vi "Create JSON Schema Interactive.vi"(8 "error in (no error)":errorcluster, 10 "Variant":variant, 11 "JSON Schema in":string) -> (0 "error out":errorcluster, 3 "JSON Schema":string)   [LabVIEW 2019, in "JSON-Schema.lvlib"]
uses:
  JSON-Schema.lvlib
  <vilib>/JDP Science/JSONtext/JSONtext.lvlib
panel:
  in  "ctl path":path
  in  "OK":bool
  in  "Table":string[][](table)
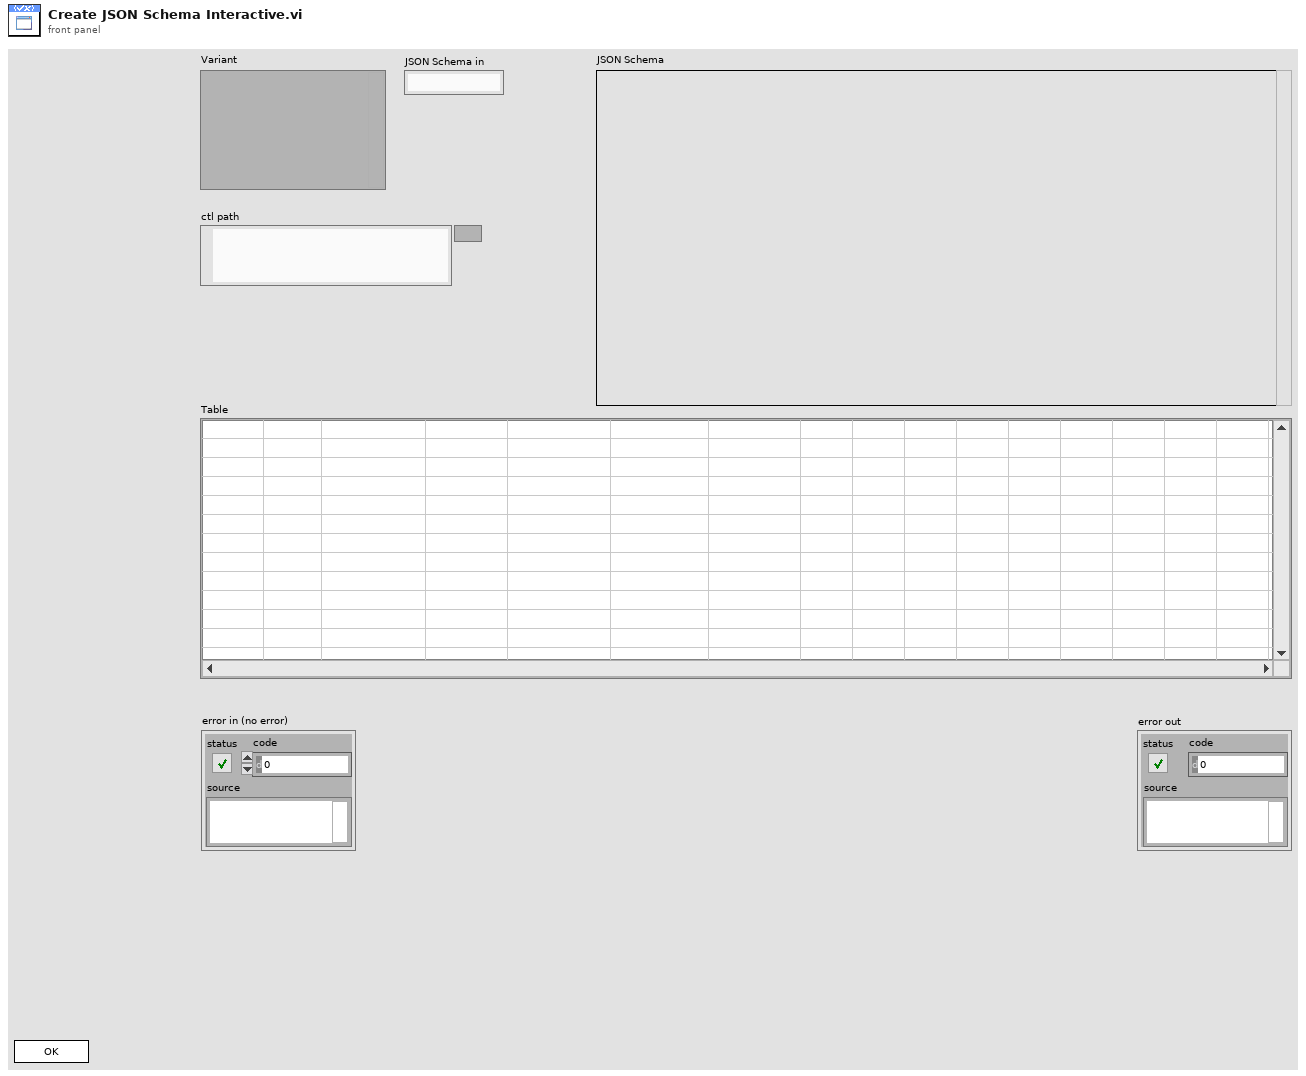
[diagram p1: front panel]
types:
  T1 = enum32{"Invalid", "Standard", "Closed", "Hidden", "Minimized", "Maximized"}
  T2 = enum32{"invalid app kind", "Development System", "Run Time System", "Student Edition", "Embedded LabVIEW", "Evaluation", "Custom"}
  T3 = cluster{"Core":cluster{"Current VI Reference":refnum<vi>, "Close Panel on Exit?":bool}, "Your Boolean data":bool, "Your string data":string}
  T4 = cluster{"Current VI Reference":refnum<vi>, "Close Panel on Exit?":bool}
  T5 = enum32{"Bad", "Idle", "Run top level", "Running"}
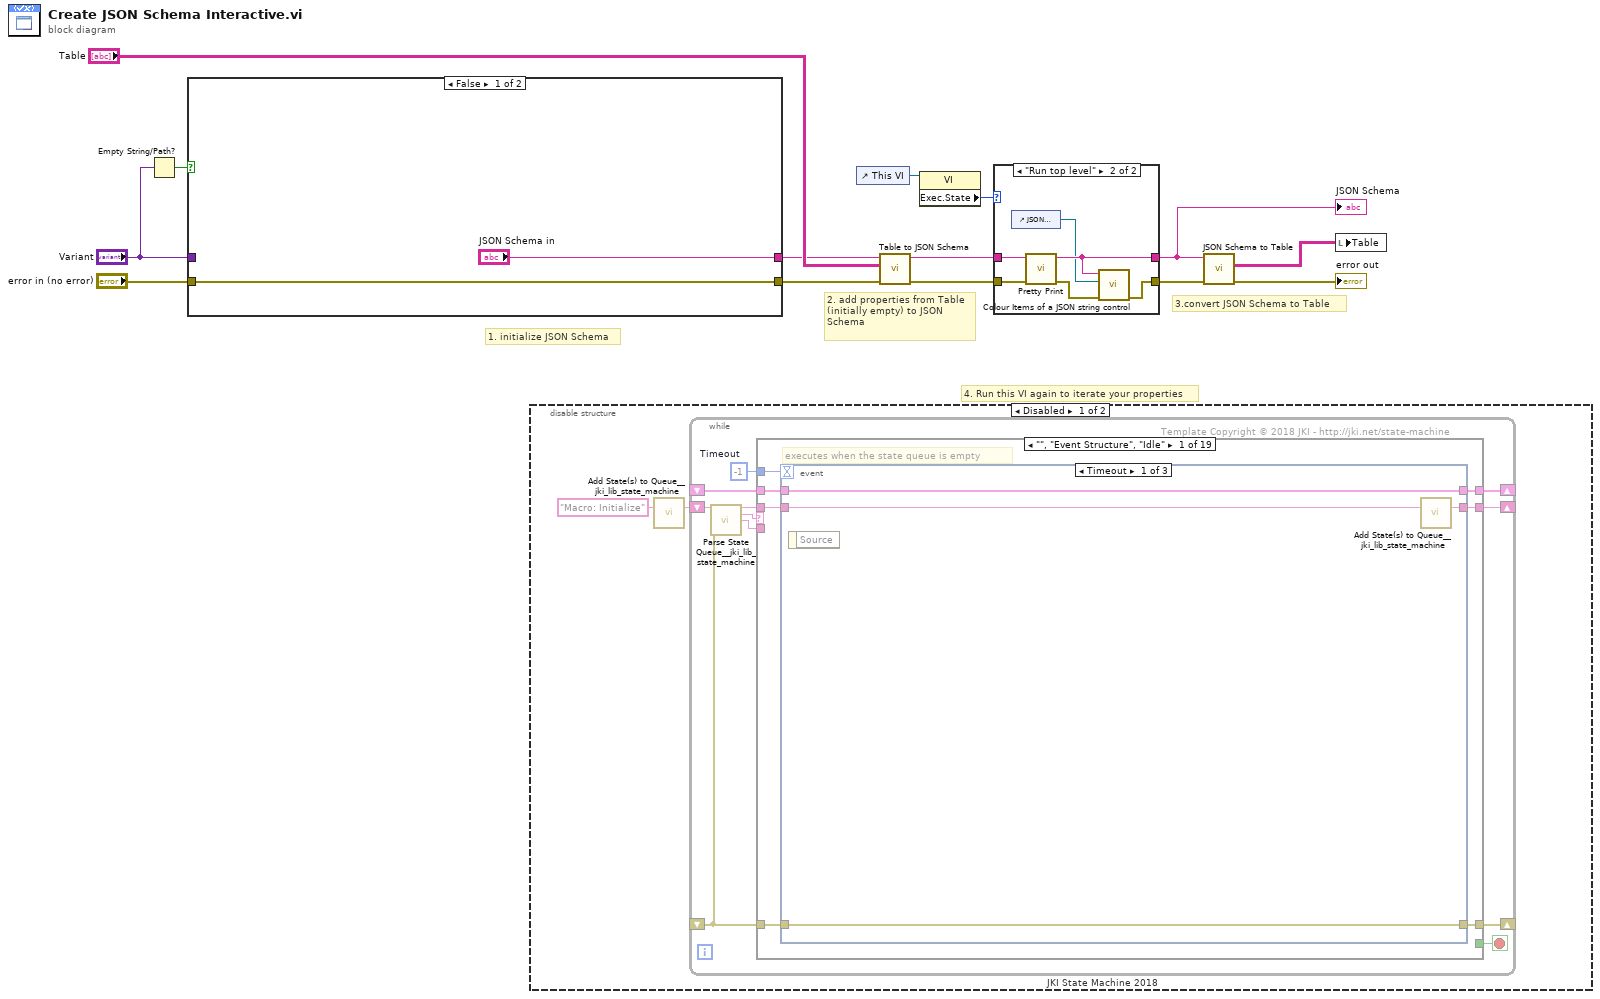
[diagram p0: block diagram]
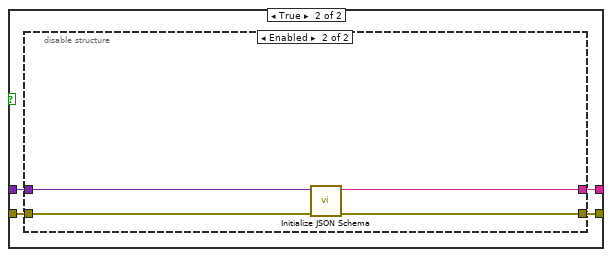
[diagram p2: hidden frame]
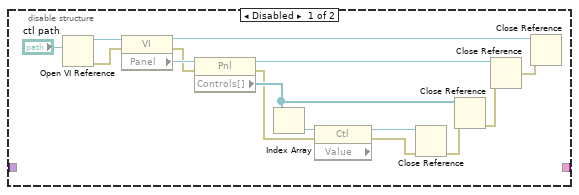
[diagram p3: hidden frame]
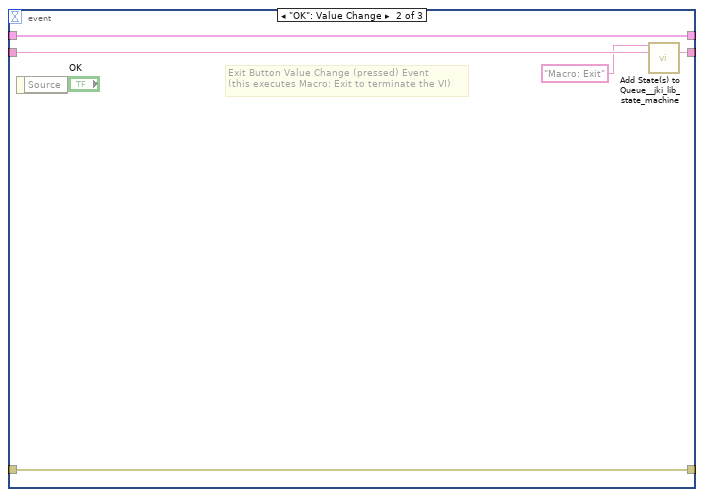
[diagram p5: hidden frame]
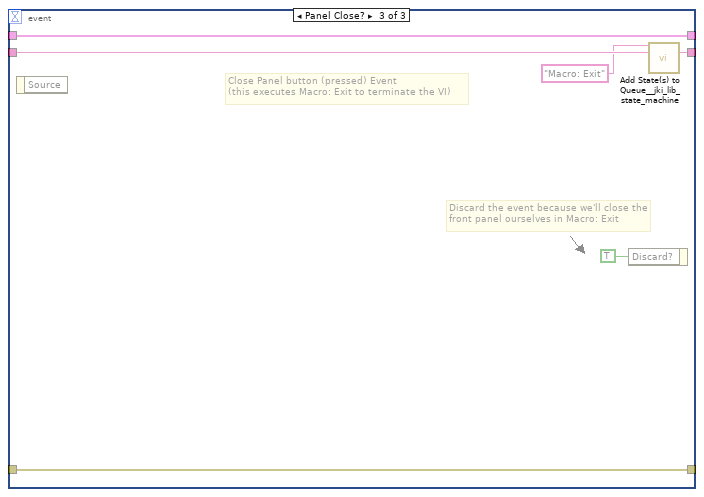
[diagram p6: hidden frame]
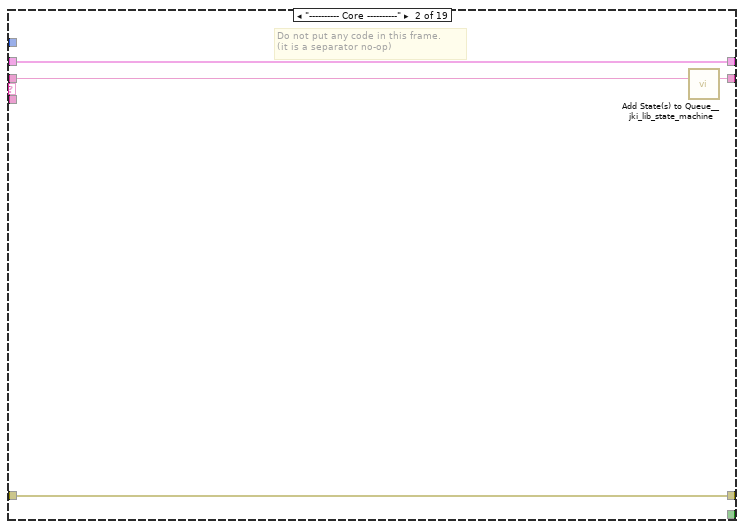
[diagram p7: hidden frame]
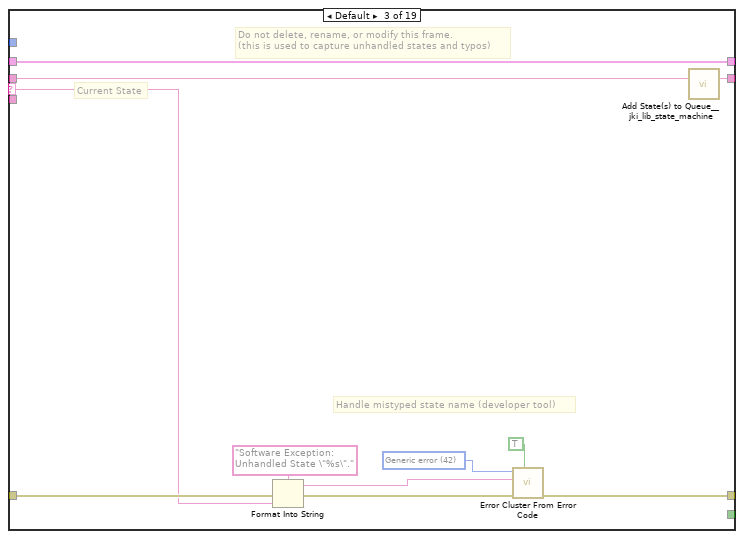
[diagram p8: hidden frame]
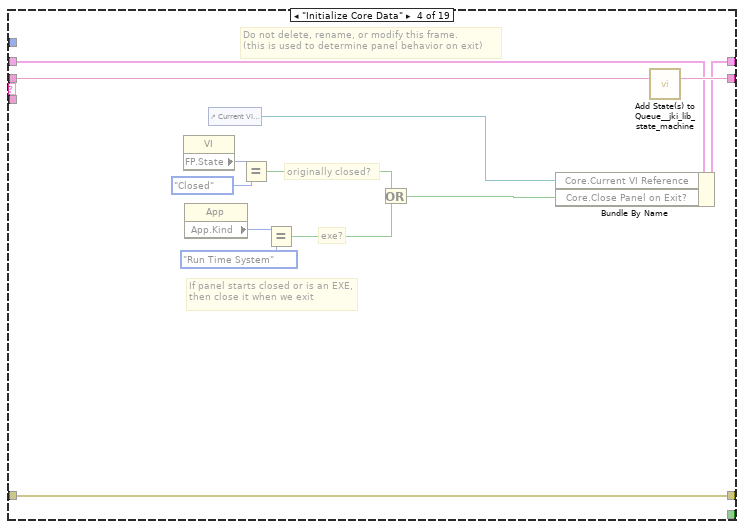
[diagram p9: hidden frame]
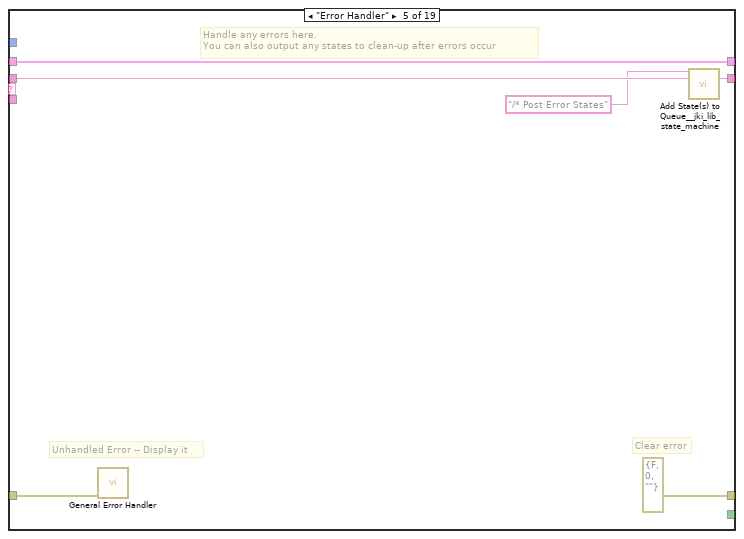
[diagram p10: hidden frame]
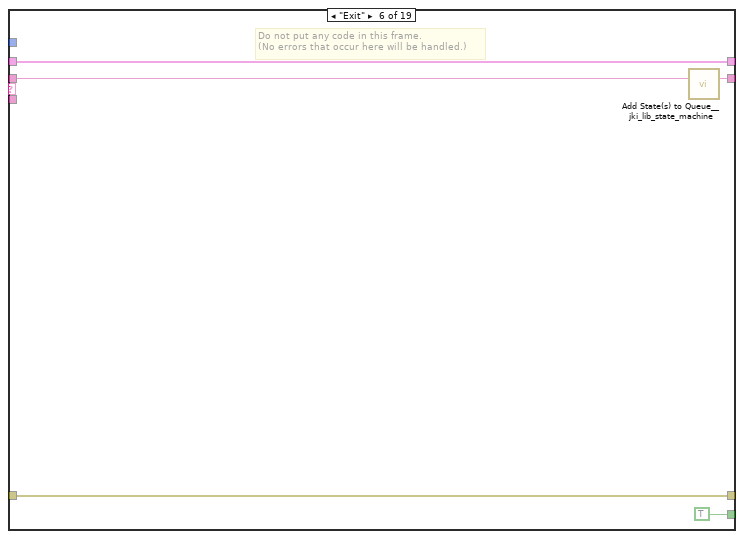
[diagram p11: hidden frame]
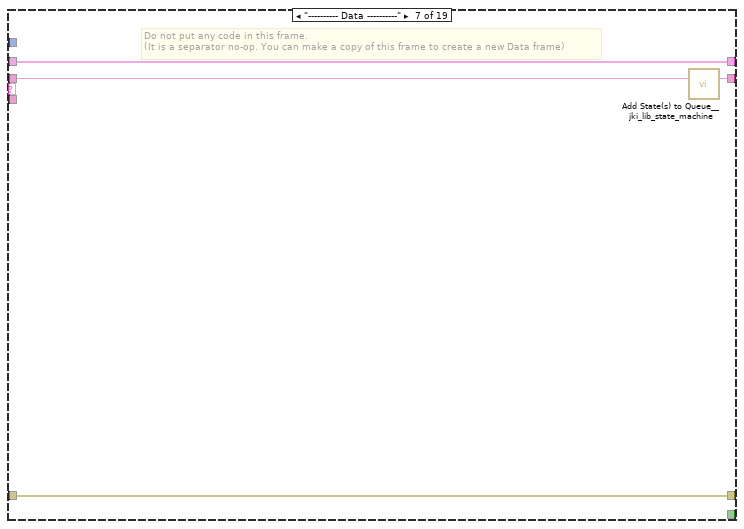
[diagram p12: hidden frame]
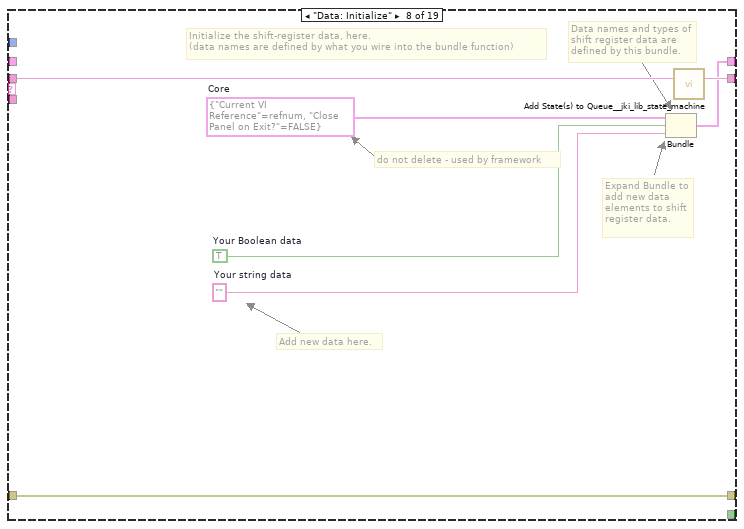
[diagram p13: hidden frame]
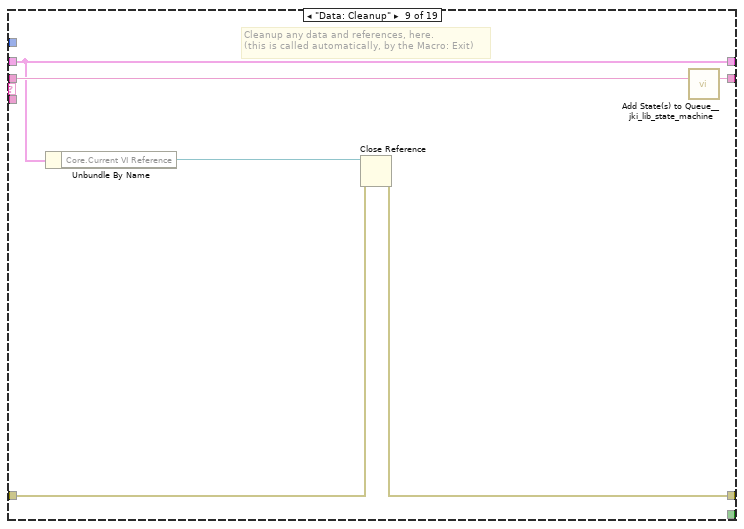
[diagram p14: hidden frame]
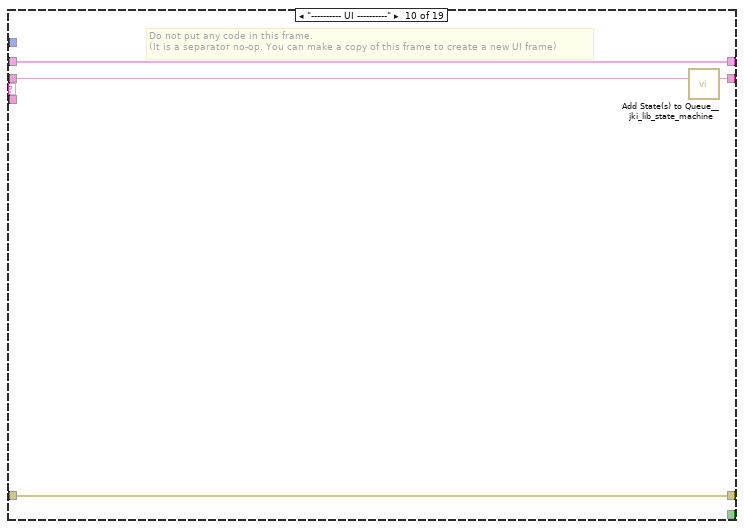
[diagram p15: hidden frame]
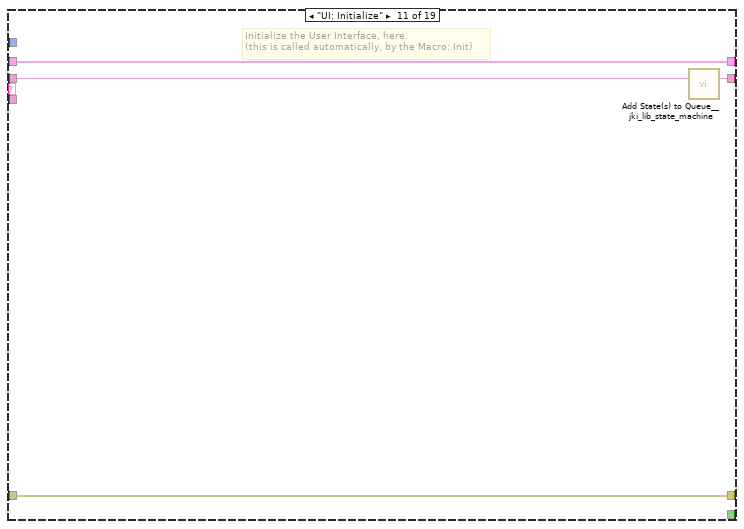
[diagram p16: hidden frame]
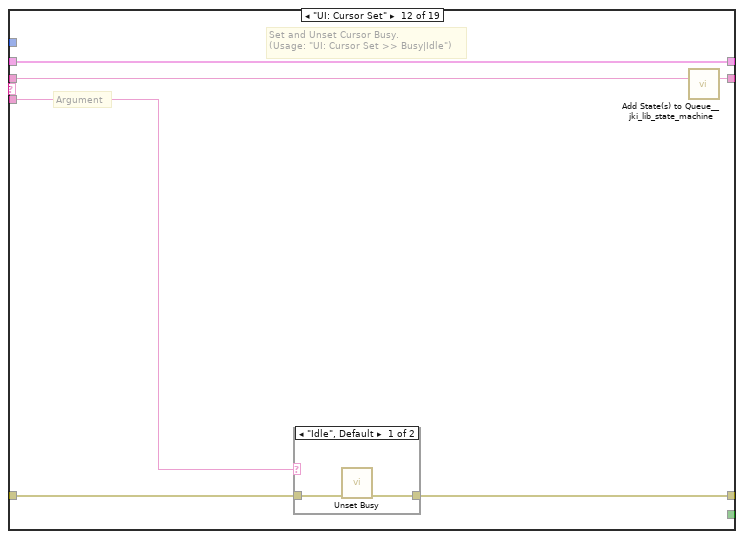
[diagram p17: hidden frame]
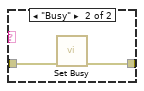
[diagram p18: hidden frame]
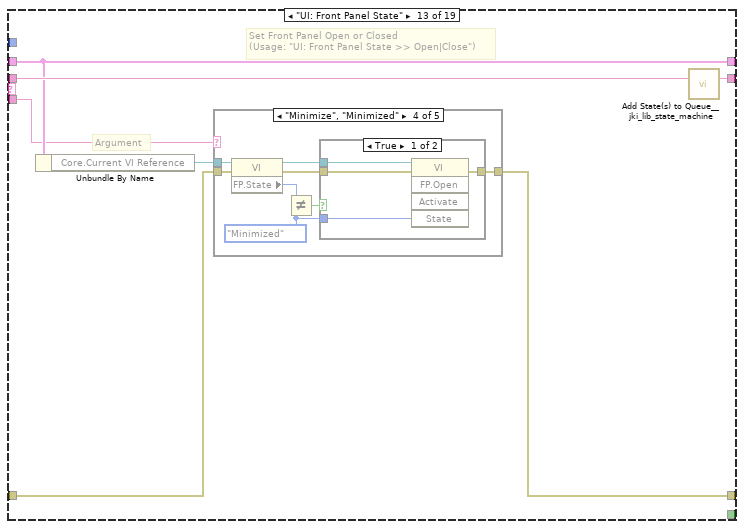
[diagram p19: hidden frame]
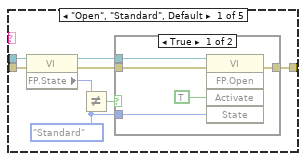
[diagram p20: hidden frame]
diagram:
  # "4. Run this VI again to iterate your properties"
  # "3.convert JSON Schema to Table"
  # "2. add properties from Table (initially empty) to JSON Schema"
  # "1. initialize JSON Schema"
  n1 = Empty String/Path?(string/path="Variant") -> (empty?=w5:bool)
  n2 = case shown="False" w5 {
    tunnel: ["JSON Schema in" w20] -> w1
    tunnel: "Variant" -> [_ w19]
    tunnel: "error in (no error)" -> [w16 w18]
    tunnel: [w16 w17] -> w2
    frame False {
    }
    frame True {
      n3 = disable-structure shown="Enabled" {
        disable-tunnel: [_ w40] -> w20
        disable-tunnel: w19 -> [_ w39]
        disable-tunnel: w18 -> [_ w38]
        disable-tunnel: [_ w37] -> w17
        frame Disabled {
          n4 = Open VI Reference(vi path="ctl path") -> (vi reference=w30:refnum<vi>, error out=w32:errorcluster)  [unwired: 5 in]
          n5 = property class="VI"(reference=w30, error in=w32) -> (reference out=w31:refnum<vi>, error out=w24:errorcluster, "Panel"=w33:refnum<vi>)
          n6 = property class="Pnl"(reference=w33, error in=w24) -> (reference out=w35:refnum<vi>, error out=w21:errorcluster, "Controls[]"=w36:refnum<vi>[])
          n7 = Index Array(array=w36) -> (element=w34:refnum<vi>)  [unwired: 1 in]
          n8 = property class="Ctl"(reference=w34, error in=w21) -> (reference out=w26:refnum<vi>, error out=w23:errorcluster, "Value"=w22:variant)
          n9 = Close Reference(reference=w26, error in (no error)=w23) -> (error out=w25:errorcluster)
          n10 = Close Reference(reference=w36, error in (no error)=w25) -> (error out=w28:errorcluster)
          n11 = Close Reference(reference=w35, error in (no error)=w28) -> (error out=w27:errorcluster)
          n12 = Close Reference(reference=w31, error in (no error)=w27) -> ()  [unwired: 1 out]
        }
        frame Enabled {
          n13 = call "Initialize JSON Schema.vi"("error in (no error)"=w38, "Variant"=w39) -> ("error out"=w37:errorcluster, "JSON Schema out"=w40:string)  [unwired: 8 in]
        }
      }
    }
  }
  n14 = disable-structure shown="Disabled" {
    frame Disabled {
      n15 = call <vilib>:"Add State(s) to Queue__jki_lib_state_machine.vi"("State(s) in (\"\")"="Macro: Initialize") -> ("States Out"=w42:string)  [unwired: 14 in]
      n16 = while "JKI State Machine 2018" {
        shift-right: [w46] -> _
        shift-left: _ -> [w45]
        shift-right: [w49] -> _
        shift-left: _ -> [w43]
        shift-right: [w48] -> _
        shift-left: w42 -> [w50]
        stop <- w47 stop-if-true
        w44 = -1  # Timeout
        # "Template Copyright © 2018 JKI - http://jki.net/state-machine"
        n17 = call <vilib>:"Parse State Queue__jki_lib_state_machine.vi"("State Queue"=w50, "Error In (no error)"=w43) -> ("Remaining States"=w52:string, "Current State"=w53:string, "Arguments"=w51:string)  [unwired: 11 in]
        n18 = case shown="\"\", \"Event Structure\", \"Idle\"" w53 {
          selector: w53 -> [_ _ w80 _ _ _ _ _ _ _ _ _ _ _ _ _ _ _ _]
          tunnel: w52 -> [w60 w79 w84 w103 w109 w114 w118 w125 w131 w135 w139 w145 w156 w225 w230 w240 w244 w248 w252]
          tunnel: w51 -> [_ _ _ _ _ _ _ _ _ _ _ w140 w150 _ _ _ _ _ _]
          tunnel: w45 -> [w58 w76 w82 w96 w106 w112 w115 _ w126 w132 w137 w143 w152 w222 w227 w237 w241 w245 w249]
          tunnel: [w57 w77 w86 w100 errorcluster {"status"=FALSE, "code"=0, "source"=""} ("error out") w111 w116 w122 w127 w133 w136 w141 w153 w223 w228 w238 w242 w246 w250] -> w49
          tunnel: w43 -> [w56 w77 w85 w100 w105 w111 w116 w122 w128 w133 w136 w142 w154 w223 w228 w238 w242 w246 w250]
          tunnel: [w59 w78 w83 w102 w108 w113 w117 w124 w130 w134 w138 w144 w155 w224 w229 w239 w243 w247 w251] -> w48
          tunnel: [_ _ _ _ _ TRUE _ _ _ _ _ _ _ _ _ _ _ _ _] -> w47
          tunnel: [w55 w76 w82 w101 w106 w112 w115 w123 w126 w132 w137 w143 w152 w222 w227 w237 w241 w245 w249] -> w46
          tunnel: w44 -> [w54 _ _ _ _ _ _ _ _ _ _ _ _ _ _ _ _ _ _]
          frame "", "Event Structure", "Idle" {
            # "executes when the state queue is empty"
            n19 = event shown="[0] Timeout" {
              selector: _ -> [_ _ _]
              dyn-events: _ -> [_ _ _]
              timeout: w54 -> [_ _ _]
              tunnel: w60 -> [w64 w69 w75]
              tunnel: [w63 w68 w74] -> w59
              tunnel: w58 -> [w61 w66 w72]
              tunnel: [w62 w67 w73] -> w57
              tunnel: w56 -> [w62 w67 w73]
              tunnel: [w61 w66 w72] -> w55
              event Timeout {
                n20 = event-data() -> ()  [unwired: 1 in, 1 out]
                n21 = call <vilib>:"Add State(s) to Queue__jki_lib_state_machine.vi"("State(s) in (\"\")"=w64) -> ("States Out"=w63:string)  [unwired: 14 in]
              }
              event "OK": Value Change {
                # "Exit Button Value Change (pressed) Event\n(this executes Macro: Exit to terminate the VI)"
                n22 = event-data() -> ()  [unwired: 1 in, 1 out]
                n23 = call <vilib>:"Add State(s) to Queue__jki_lib_state_machine.vi"("State(s) in Front (\"\")"="Macro: Exit", "State(s) in (\"\")"=w69) -> ("States Out"=w68:string)  [unwired: 13 in]
              }
              event Panel Close? {
                # "Discard the event because we'll close the front panel ourselves in Macro: Exit"
                # "Close Panel button (pressed) Event\n(this executes Macro: Exit to terminate the VI)"
                n24 = event-data() -> ()  [unwired: 1 in, 1 out]
                n25 = event-data("Discard?"=TRUE) -> ()  [unwired: 1 in, 1 out]
                n26 = call <vilib>:"Add State(s) to Queue__jki_lib_state_machine.vi"("State(s) in Front (\"\")"="Macro: Exit", "State(s) in (\"\")"=w75) -> ("States Out"=w74:string)  [unwired: 13 in]
              }
            }
          }
          frame "---------- Core ----------" {
            # "Do not put any code in this frame.\n(it is a separator no-op)"
            n27 = call <vilib>:"Add State(s) to Queue__jki_lib_state_machine.vi"("State(s) in (\"\")"=w79) -> ("States Out"=w78:string)  [unwired: 14 in]
          }
          frame Default {
            w89 = 42 items=["No error", "Argument error", "Memory is full", "Out of zone", "End of file", "File already open", "Generic file I/O error", "File not found", "File permission error", "Disk is full", "Duplicate path", "Too many files open", "System feature not enabled", "Resource file not found", "Cannot add resource", "Resource not found", "Image not found", "Image memory error", "Pen does not exist", "Config type invalid", "Config token not found", "Config parse error", "Config memory error", "Bad external code format", "Bad external code offset", "External code not present", "Null window", "Destroy window error", "Null menu", "Print aborted", "Bad print record", "Print driver error", "Windows error during printing", "Memory error during printing", "Print dialog error", "Generic print error", "Invalid device refnum", "Device not found", "Device parameter error", "Device unit error", "Cannot open device", "Device call aborted", "Generic error", "Cancelled by user", "Object ID too low", "Object ID too high", "Object not in heap", "Unknown heap", "Unknown object (invalid DefProc)", "Unknown object (DefProc not in table)", "Message out of range", "Invalid (null) method", "Unknown message", "Manager call not supported", "Bad address", "Network operation in progress", "Network operation timed out", "Connection is busy", "Network attribute not supported", "Network error", "Address in use", "System out of memory", "Connection aborted", "Connection refused", "Not connected", "Already connected", "Connection closed", "Initialization error (interapplication manager)", "Bad occurrence", "Wait on unbound occurrence handler", "Occurrence queue overflow", "Datalog type conflict", "Unused", "Unrecognized type (interapplication manager)", "Memory corrupt", "Failed to make temporary DLL", "Old CIN version", "Drag socket not found", "Failed to load drop-object", "Failed to register OLE object", "Failed to release OLE object", "Format specifier type mismatch", "Unknown format specifier", "Too few format specifiers", "Too many format specifiers", "Scan failed", "Newer CIN version", "Error converting to variant", "Runtime menu error", "Password tampered", "Variant attribute not found", "Incompatible variant data type", "Event data is not available", "Event Store is not present", "Occurrence is not found", "Event Queue is not created", "Event info is not available", "Refnum passed is NULL", "Error retrieving Class GUID", "Error retrieving CoClass GUID", "Error retrieving TypeLib GUID.", "Bad built application magic bytes.", "Specific driver is different from the specific driver associated with the Logical Name.", "There is no session opened to the class driver.", "Max Error", "MAX - Error with config objects", "MAX - Error loading configuration", "MAX - Group not supported"]
            # "Current State"
            # "Do not delete, rename, or modify this frame.\n(this is used to capture unhandled states and typos)"
            # "Handle mistyped state name (developer tool)"
            n28 = Format Into String(format string="Software Exception: Unhandled State \"%s\"." ("message"), error in=w85, w80) -> (resulting string=w88:string, error out=w87:errorcluster)  [unwired: 1 in]
            n29 = call <vilib>:"Error Cluster From Error Code.vi"("show call chain? (False)"=TRUE, "error in (no error)"=w87, "error message (\"\")"=w88, "error code (0)"=w89) -> ("error out"=w86:errorcluster)  [unwired: 5 in]
            n30 = call <vilib>:"Add State(s) to Queue__jki_lib_state_machine.vi"("State(s) in (\"\")"=w84) -> ("States Out"=w83:string)  [unwired: 14 in]
          }
          frame "Initialize Core Data" {
            # "Do not delete, rename, or modify this frame.\n(this is used to determine panel behavior on exit)"
            # "originally closed?"
            # "exe?"
            # "If panel starts closed or is an EXE, then close it when we exit"
            n31 = property class="VI"() -> ("FP.State"=w93:T1)  [unwired: 2 in, 2 out]
            n32 = property class="App"() -> ("App.Kind"=w99:T2)  [unwired: 2 in, 2 out]
            n33 = control-ref of="Current VI Reference"() -> (w94:refnum<vi>)
            n34 = Equal?(x=w93, y=T1."Closed" ("Front Panel Window:State")) -> (x = y?=w91:bool)
            n35 = Equal?(x=w99, y=T2."Run Time System" ("Application:Kind")) -> (x = y?=w97:bool)
            n36 = Or(x=w91, y=w97) -> (x .or. y?=w95:bool)
            n37 = Bundle By Name(cluster=w96, "Core.Current VI Reference"=w94, "Core.Close Panel on Exit?"=w95) -> (w101:T3)
            n38 = call <vilib>:"Add State(s) to Queue__jki_lib_state_machine.vi"("State(s) in (\"\")"=w103) -> ("States Out"=w102:string)  [unwired: 14 in]
          }
          frame "Error Handler" {
            # "Unhandled Error -- Display it"
            # "Handle any errors here.\nYou can also output any states to clean-up after errors occur"
            # "Clear error"
            n39 = call <vilib>:"General Error Handler.vi"("error in (no error)"=w105) -> ()  [unwired: 10 in, 5 out]
            n40 = call <vilib>:"Add State(s) to Queue__jki_lib_state_machine.vi"("State(s) in Front (\"\")"="/* Post Error States", "State(s) in (\"\")"=w109) -> ("States Out"=w108:string)  [unwired: 13 in]
          }
          frame "Exit" {
            # "Do not put any code in this frame.\n(No errors that occur here will be handled.)"
            n41 = call <vilib>:"Add State(s) to Queue__jki_lib_state_machine.vi"("State(s) in (\"\")"=w114) -> ("States Out"=w113:string)  [unwired: 14 in]
          }
          frame "---------- Data ----------" {
            # "Do not put any code in this frame.\n(It is a separator no-op. You can make a copy of this frame to create a new Data frame)"
            n42 = call <vilib>:"Add State(s) to Queue__jki_lib_state_machine.vi"("State(s) in (\"\")"=w118) -> ("States Out"=w117:string)  [unwired: 14 in]
          }
          frame "Data: Initialize" {
            w119 = T4 {"Current VI Reference"=refnum, "Close Panel on Exit?"=FALSE}  # Core
            w121 = TRUE  # Your Boolean data
            w120 = ""  # Your string data
            # "do not delete - used by framework"
            # "Expand Bundle to add new data elements to shift register data."
            # "Add new data here."
            # "Data names and types of shift register data are defined by this bundle."
            # "Initialize the shift-register data, here.\n(data names are defined by what you wire into the bundle function)"
            n43 = Bundle("Core"=w119, "Your Boolean data"=w121, "Your string data"=w120) -> (w123:T3)  [unwired: 1 in]
            n44 = call <vilib>:"Add State(s) to Queue__jki_lib_state_machine.vi"("State(s) in (\"\")"=w125) -> ("States Out"=w124:string)  [unwired: 14 in]
          }
          frame "Data: Cleanup" {
            # "Cleanup any data and references, here.\n(this is called automatically, by the Macro: Exit)"
            n45 = Unbundle By Name(w126) -> ("Core.Current VI Reference"=w129:refnum<vi>)
            n46 = Close Reference(reference=w129, error in (no error)=w128) -> (error out=w127:errorcluster)
            n47 = call <vilib>:"Add State(s) to Queue__jki_lib_state_machine.vi"("State(s) in (\"\")"=w131) -> ("States Out"=w130:string)  [unwired: 14 in]
          }
          frame "---------- UI ----------" {
            # "Do not put any code in this frame.\n(It is a separator no-op. You can make a copy of this frame to create a new UI frame)"
            n48 = call <vilib>:"Add State(s) to Queue__jki_lib_state_machine.vi"("State(s) in (\"\")"=w135) -> ("States Out"=w134:string)  [unwired: 14 in]
          }
          frame "UI: Initialize" {
            # "Initialize the User Interface, here.\n(this is called automatically, by the Macro: Init)"
            n49 = call <vilib>:"Add State(s) to Queue__jki_lib_state_machine.vi"("State(s) in (\"\")"=w139) -> ("States Out"=w138:string)  [unwired: 14 in]
          }
          frame "UI: Cursor Set" {
            # "Argument"
            # "Set and Unset Cursor Busy.\n(Usage: \"UI: Cursor Set >> Busy|Idle\")"
            n50 = case shown="\"Idle\", Default" w140 {
              tunnel: w142 -> [w147 w149]
              tunnel: [w146 w148] -> w141
              frame "Idle", Default {
                n51 = call <vilib>:"Unset Busy.vi"("error in (no error)"=w147) -> ("error out"=w146:errorcluster)  [unwired: 10 in]
              }
              frame "Busy" {
                n52 = call <vilib>:"Set Busy.vi"("error in (no error)"=w149) -> ("error out"=w148:errorcluster)  [unwired: 9 in, 1 out]
              }
            }
            n53 = call <vilib>:"Add State(s) to Queue__jki_lib_state_machine.vi"("State(s) in (\"\")"=w145) -> ("States Out"=w144:string)  [unwired: 14 in]
          }
          frame "UI: Front Panel State" {
            # "Argument"
            # "Set Front Panel Open or Closed\n(Usage: \"UI: Front Panel State >> Open|Close\")"
            n54 = Unbundle By Name(w152) -> ("Core.Current VI Reference"=w151:refnum<vi>)
            n55 = case shown="\"Minimize\", \"Minimized\"" w150 {
              tunnel: w154 -> [w162 w177 w188 w201 w214]
              tunnel: [w164 w178 w190 w203 w216] -> w153
              tunnel: w151 -> [w163 w175 w189 w202 w215]
              frame "Open", "Standard", Default {
                w157 = T1."Standard" ("State")
                n56 = property class="VI"(reference=w163, error in=w162) -> (reference out=w160:refnum<vi>, error out=w161:errorcluster, "FP.State"=w159:T1)
                n57 = Not Equal?(x=w159, y=w157) -> (x != y?=w158:bool)
                n58 = case shown="True" w158 {
                  tunnel: [w168 w170] -> w164
                  tunnel: w161 -> [w167 w170]
                  tunnel: w160 -> [w166 _]
                  tunnel: w157 -> [w165 _]
                  frame True {
                    n59 = invoke class="VI" method="FP.Open"(reference=w166, error in=w167, "Activate"=TRUE, "State"=w165) -> (error out=w168:errorcluster)  [unwired: 1 in, 4 out]
                  }
                  frame False {
                  }
                }
              }
              frame "Close", "Closed" {
                n60 = property class="VI"(reference=w175, error in=w177) -> (reference out=w174:refnum<vi>, error out=w176:errorcluster, "FP.State"=w172:T1)
                n61 = Not Equal?(x=w172, y=T1."Closed" ("Front Panel Window:State")) -> (x != y?=w171:bool)
                n62 = case shown="True" w171 {
                  tunnel: [w179 w182] -> w178
                  tunnel: w176 -> [w179 w181]
                  tunnel: w174 -> [_ w180]
                  frame False {
                  }
                  frame True {
                    n63 = invoke class="VI" method="FP.Close"(reference=w180, error in=w181) -> (error out=w182:errorcluster)  [unwired: 1 in, 2 out]
                  }
                }
              }
              frame "Hidden", "Hide" {
                w183 = T1."Hidden" ("State")
                n64 = property class="VI"(reference=w189, error in=w188) -> (reference out=w186:refnum<vi>, error out=w187:errorcluster, "FP.State"=w185:T1)
                n65 = Not Equal?(x=w185, y=w183) -> (x != y?=w184:bool)
                n66 = case shown="True" w184 {
                  tunnel: [w194 w195] -> w190
                  tunnel: w187 -> [w193 w195]
                  tunnel: w186 -> [w192 _]
                  tunnel: w183 -> [w191 _]
                  frame True {
                    n67 = invoke class="VI" method="FP.Open"(reference=w192, error in=w193, "State"=w191) -> (error out=w194:errorcluster)  [unwired: 2 in, 4 out]
                  }
                  frame False {
                  }
                }
              }
              frame "Minimize", "Minimized" {
                w196 = T1."Minimized" ("State")
                n68 = property class="VI"(reference=w202, error in=w201) -> (reference out=w199:refnum<vi>, error out=w200:errorcluster, "FP.State"=w198:T1)
                n69 = Not Equal?(x=w198, y=w196) -> (x != y?=w197:bool)
                n70 = case shown="True" w197 {
                  tunnel: [w207 w208] -> w203
                  tunnel: w200 -> [w206 w208]
                  tunnel: w199 -> [w205 _]
                  tunnel: w196 -> [w204 _]
                  frame True {
                    n71 = invoke class="VI" method="FP.Open"(reference=w205, error in=w206, "State"=w204) -> (error out=w207:errorcluster)  [unwired: 2 in, 4 out]
                  }
                  frame False {
                  }
                }
              }
              frame "Maximize", "Maximized" {
                w209 = T1."Maximized" ("State")
                n72 = property class="VI"(reference=w215, error in=w214) -> (reference out=w212:refnum<vi>, error out=w213:errorcluster, "FP.State"=w211:T1)
                n73 = Not Equal?(x=w211, y=w209) -> (x != y?=w210:bool)
                n74 = case shown="True" w210 {
                  tunnel: [w220 w221] -> w216
                  tunnel: w213 -> [w219 w221]
                  tunnel: w212 -> [w218 _]
                  tunnel: w209 -> [w217 _]
                  frame True {
                    n75 = invoke class="VI" method="FP.Open"(reference=w218, error in=w219, "State"=w217) -> (error out=w220:errorcluster)  [unwired: 2 in, 4 out]
                  }
                  frame False {
                  }
                }
              }
            }
            n76 = call <vilib>:"Add State(s) to Queue__jki_lib_state_machine.vi"("State(s) in (\"\")"=w156) -> ("States Out"=w155:string)  [unwired: 14 in]
          }
          frame "---------- Macro ----------" {
            # "Do not put any code in this frame.\n(It is a separator no-op. You can make a copy of this frame to create a new Macro frame)"
            n77 = call <vilib>:"Add State(s) to Queue__jki_lib_state_machine.vi"("State(s) in (\"\")"=w225) -> ("States Out"=w224:string)  [unwired: 14 in]
          }
          frame "Macro: Initialize" {
            w226 = "Data: Initialize\nInitialize Core Data\nUI: Initialize\nUI: Front Panel State >> Open"  # Data: Initialize Initialize Core Data UI: Initialize UI: Front Panel State >> Open
            # "Initialization Macro\n(This is called once, when the VI starts)"
            n78 = call <vilib>:"Add State(s) to Queue__jki_lib_state_machine.vi"("State(s) in Front (\"\")"=w226, "State(s) in (\"\")"=w230) -> ("States Out"=w229:string)  [unwired: 13 in]
          }
          frame "Macro: Exit" {
            # "Exit Macro\n(This is called once, when the VI exits)"
            n79 = Unbundle By Name(w237) -> ("Core.Close Panel on Exit?"=w236:bool)
            n80 = Select(t="UI: Front Panel State >> Close", s=w236, f="") -> (s? t:f=w233:string)
            n81 = call <vilib>:"Add State(s) to Queue__jki_lib_state_machine.vi"("State(s) in (\"\")"=w233, "State(s) at Back (\"\")"="Data: Cleanup\nExit") -> ("States Out"=w231:string)  [unwired: 13 in]
            n82 = call <vilib>:"Add State(s) to Queue__jki_lib_state_machine.vi"("State(s) in Front (\"\")"=w231, "State(s) in (\"\")"=w240) -> ("States Out"=w239:string)  [unwired: 13 in]
          }
          frame "---------- New Category ----------" {
            # "Template Separator\n(You can make a copy of, or modify, this frame)"
            n83 = call <vilib>:"Add State(s) to Queue__jki_lib_state_machine.vi"("State(s) in (\"\")"=w244) -> ("States Out"=w243:string)  [unwired: 14 in]
          }
          frame "New Category: 1" {
            # "Your code here.\n(You can make a copy of, or modify, this frame)"
            n84 = call <vilib>:"Add State(s) to Queue__jki_lib_state_machine.vi"("State(s) in (\"\")"=w248) -> ("States Out"=w247:string)  [unwired: 14 in]
          }
          frame "New Category: 2" {
            # "Your code here.\n(You can make a copy of, or modify, this frame)"
            n85 = call <vilib>:"Add State(s) to Queue__jki_lib_state_machine.vi"("State(s) in (\"\")"=w252) -> ("States Out"=w251:string)  [unwired: 14 in]
          }
        }
      }
    }
    frame Enabled {
    }
  }
  n86 = control-ref of="This VI"() -> (w14:refnum<vi>)
  n87 = call "Table to JSON Schema.vi"("error in (no error)"=w2, "Table"="Table", "JSON Schema in"=w1) -> ("error out"=w11:errorcluster, "JSON Schema out"=w12:string)  [unwired: 7 in]
  n88 = property class="VI"(reference=w14) -> ("Exec.State"=w13:T5)  [unwired: 1 in, 2 out]
  n89 = case shown="\"Run top level\"" w13 {
    tunnel: w12 -> [w253 w260]
    tunnel: w11 -> [w254 w259]
    tunnel: [w254 w255] -> w10
    tunnel: [w253 w258] -> w6
    frame Default {
    }
    frame "Run top level" {
      n90 = control-ref of="JSON Schema"() -> (w257:refnum<vi>)
      n91 = call <vilib>:"Pretty Print.vi"("error in (no error)"=w259, "JSON"=w260) -> ("error out"=w256:errorcluster, "<JSON>"=w258:string)  [unwired: 7 in, 1 out]
      n92 = call <vilib>:"Colour Items of a JSON string control.vi"("error in (no error)"=w256, "String Control"=w257, "JSON"=w258) -> ("error out"=w255:errorcluster)  [unwired: 8 in]
    }
  }
  "JSON Schema" <- w6
  n93 = call "JSON Schema to Table.vi"("error in (no error)"=w10, "JSON Schema in"=w6) -> ("error out"=→"error out":errorcluster, "Table"=w8:string[][])  [unwired: 8 in]
  n94 = local write "Table"(w8) -> ()
